vi "Write To SS w error io.vi"(0 "file path (dialog if empty)":path, 3 "format (%.3f)":string="%.3f", 7 "2D data":dbl[][](array[numeric]) format="%0.2f", 9 "1D data":dbl[](array[numeric]) format="%0.2f", 11 "error in":errorcluster, 12 "append to file? (new file:F)":bool, 13 "transpose? (no:F)":bool, 14 "delimiter (\\t)":string="\t") -> (4 "new file path (Not A Path if cancelled)":path, 15 "error out":errorcluster)   [LabVIEW 2014]
doc: "Converts a 2D or 1D array of single-precision numbers to a text string and writes the string to a new byte stream file or appends the string to an existing file.\n\nmodified to allow error\n\nPaul K Dixon\nPhysics 350\nCSUSB Physics"
panel:
  in  "prompt":string="Choose file to write."
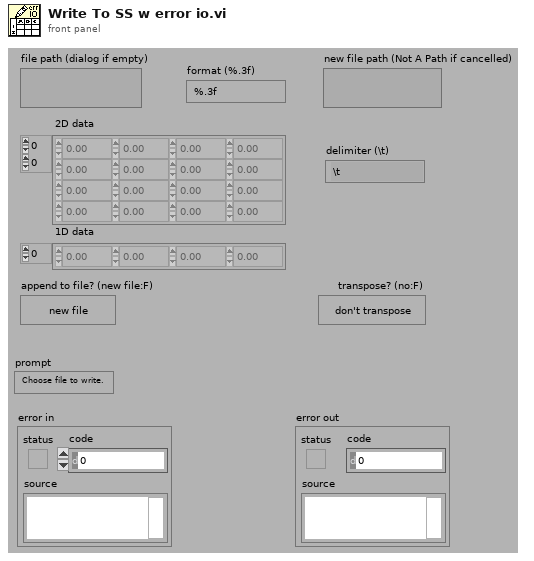
[diagram p1: front panel]
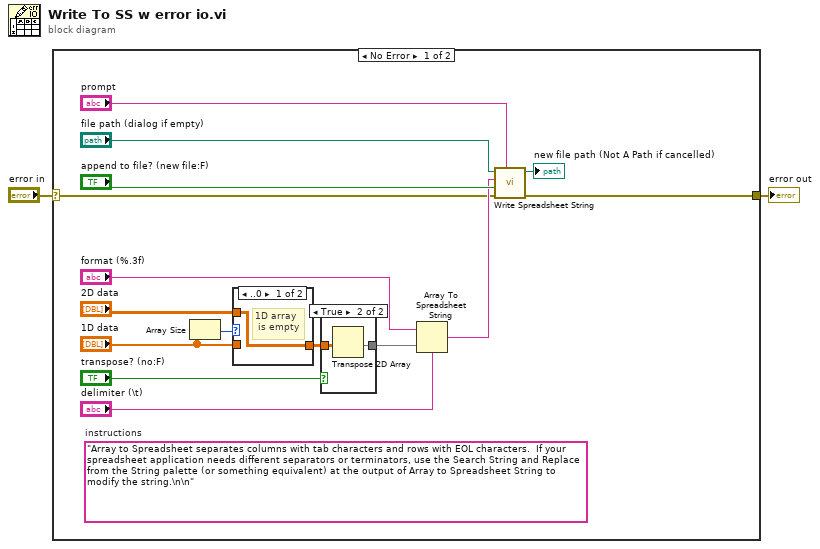
[diagram p0: block diagram]
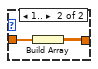
[diagram p3: hidden frame]
diagram:
  n1 = case shown="No Error" "error in" {
    selector: "error in" -> [w3 w24]
    tunnel: [w4 w24] -> w2
    frame No Error {
      (unwired) "Array to Spreadsheet separates columns with tab characters and rows with EOL characters.  If your spreadsheet application needs different separators or terminators, use the Search String and Replace from the String palette (or something equivalent) at the output of Array to Spreadsheet String to modify the string.\n\n"  # instructions
      n2 = Array Size(array="1D data") -> (size(s)=w16:i32)
      n3 = case shown="..0" w16 {
        tunnel: "1D data" -> [_ w23]
        tunnel: [w21 w22] -> w12
        tunnel: "2D data" -> [w21 _]
        frame ..0 {
          # "1D array\n is empty"
        }
        frame 1.. {
          n4 = Build Array(w23) -> (w22:dbl[][])
        }
      }
      n5 = case shown="True" "transpose? (no:F)" {
        tunnel: [w18 w20] -> w10
        tunnel: w12 -> [w18 w19]
        frame False {
        }
        frame True {
          n6 = Transpose 2D Array(2D array=w19) -> (transposed array=w20:dbl[][])
        }
      }
      n7 = Array To Spreadsheet String(delimiter (Tab)="delimiter (\\t)", array=w10, 3:"format (%.3f)") -> (spreadsheet string=w5:string)
      n8 = call <vilib>:"Write Spreadsheet String.vi"("prompt"="prompt", "error in"=w3, "append to file? (new file:F)"="append to file? (new file:F)", "spreadsheet string"=w5, "file path (dialog if empty)"="file path (dialog if empty)") -> ("error out"=w4:errorcluster, "path"=→"new file path (Not A Path if cancelled)":path)  [unwired: 2 in, 3 out]
    }
    frame Error {
    }
  }
  "error out" <- w2
